vi "destroy.vi"(8 "error in":errorcluster, 11 "task token in":refnum<class "null task token.lvclass">) -> (0 "error out":errorcluster)   [LabVIEW 2013, in "null task token.lvclass"]
uses:
  null task token.lvclass
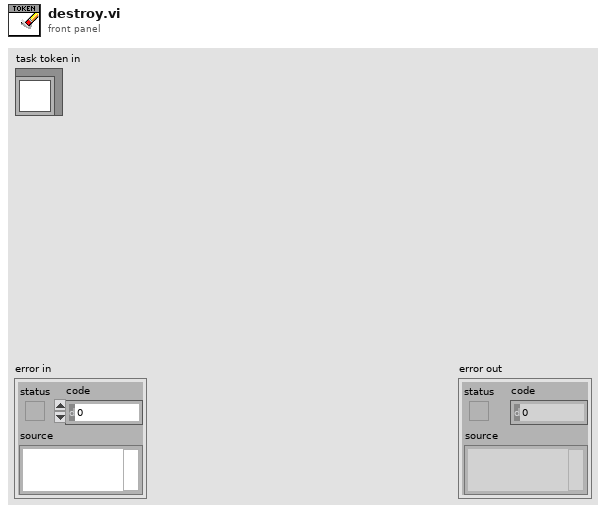
[diagram p1: front panel]
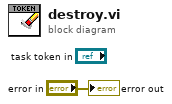
[diagram p0: block diagram]
diagram:
  "error out" <- "error in"
